vi "Result_Test.vi"(8 "error in (no error)":errorcluster caption="entrée d'erreur (pas d'erreur)", 11 "Delay en entrée":refnum<class "Enter_Batch.lvclass">) -> (0 "error out":errorcluster caption="sortie d'erreur", 3 "Delay en sortie":refnum<class "Enter_Batch.lvclass">)   [LabVIEW 2020, in "Library Test.lvlib" / "Enter_Batch.lvclass"]
uses:
  Enter_Batch.lvclass
  C:/Users/ngarcin/OneDrive - Altyor/Standard TB/Class/Test/Test (Default)/Test (Default).lvclass
  Test_Without_Instr/Test_Without_Inst.lvclass
  Enter_Batch.lvclass/Enter_Batch.ctl
  Commun VI/Library Commun.lvlib
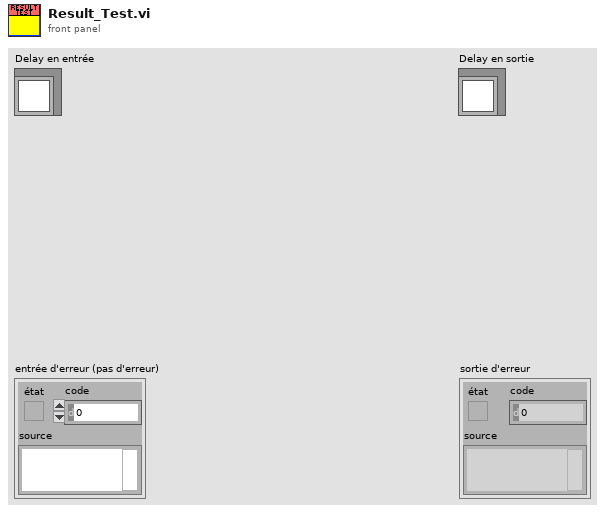
[diagram p1: front panel]
types:
  T1 = enum16{"Get Variable", "Get All Variables", "Set Variable", "Delete Variable", "Delete All Variable"}
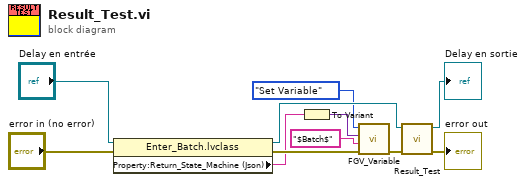
[diagram p0: block diagram]
diagram:
  n1 = property class="Enter_Batch.lvclass"(reference="Delay en entrée", error in="error in (no error)") -> (reference out=w8:refnum<class "Enter_Batch.lvclass">, error out=w6:errorcluster, "Property:Return_State_Machine (Json)"=w4:string)
  n2 = To Variant(anything=w4) -> (Variant=w2:variant)
  n3 = call "FGV_Variable.vi"("error in (no error)"=w6, "Variable"="$Batch$" ("Name"), "Data In"=w2, "Function"=T1."Set Variable") -> ("error out"=w5:errorcluster)  [unwired: 5 in, 2 out]
  n4 = call-parent "Result_Test.vi"("error in (no error)"=w5, "Test_Without_Inst en entrée"=w8) -> ("error out"=→"error out":errorcluster, "Test_Without_Inst en sortie"=→"Delay en sortie":refnum<class "Enter_Batch.lvclass">)  [unwired: 8 in]
